vi "Filter Default message.vi"(6 "Default 3":string, 7 "new element/subarray":string[](array[string]), 8 "Default 2":string, 9 "Default 1":string, 11 "CAN TABLE":string[][](array[string])) -> (3 "CAN TABLE 2":string[][](array[string]))   [LabVIEW 2017]
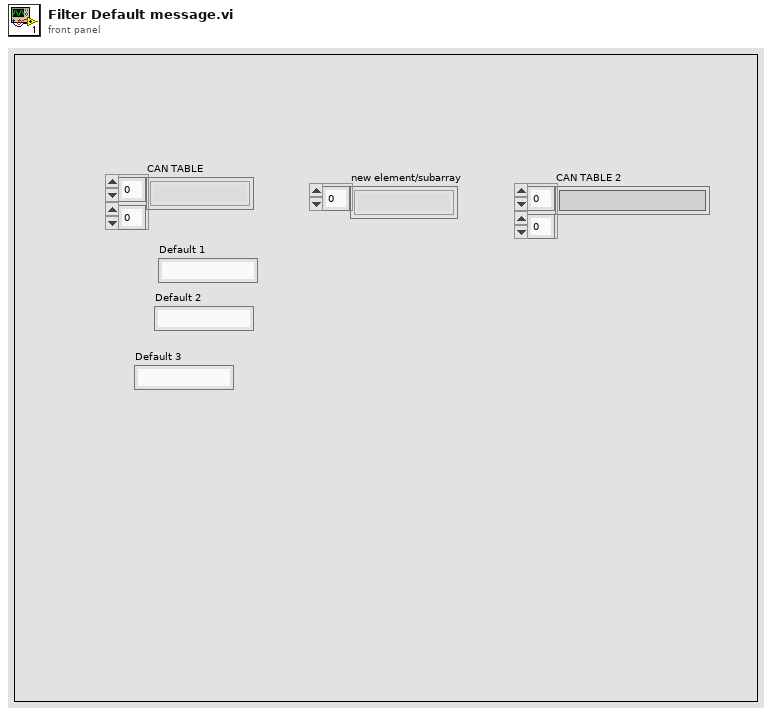
[diagram p1: front panel]
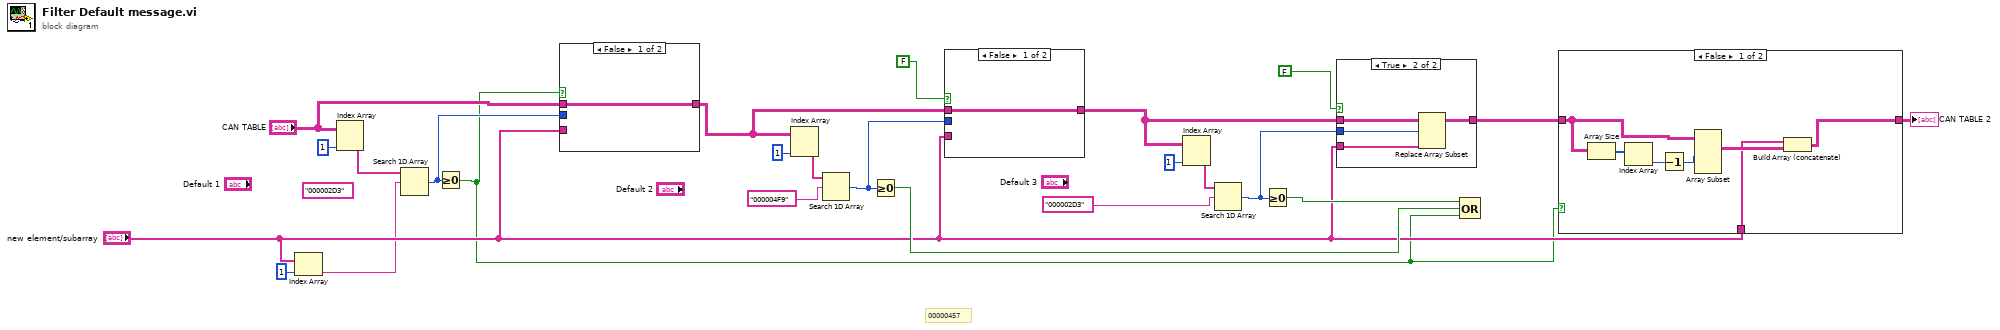
[diagram p0: block diagram]
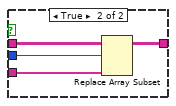
[diagram p4: hidden frame]
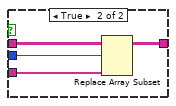
[diagram p5: hidden frame]
diagram:
  (unwired) "000002D3" ("element")
  # "00000457"
  n1 = Index Array(array="new element/subarray", index=1) -> (element=w4:string)
  n2 = Index Array(array="CAN TABLE", index (col)=1 ("disabled index (col)")) -> (element=w23:string[])  [unwired: 1 in]
  n3 = Search 1D Array(1D array=w23, element=w4) -> (index of element=w22:i32)  [unwired: 1 in]
  n4 = Greater Or Equal To 0?(x=w22) -> (x >= 0?=w1:bool)
  n5 = case shown="False" w1 {
    tunnel: w22 -> [_ w29]
    tunnel: [w25 w28] -> w18
    tunnel: "CAN TABLE" -> [w25 w27]
    tunnel: "new element/subarray" -> [_ w26]
    frame False {
    }
    frame True {
      n6 = Replace Array Subset(array=w27, new element=w26, index (row)=w29) -> (w28:string[][])  [unwired: 1 in]
    }
  }
  n7 = Index Array(array=w18, index (col)=1 ("disabled index (col)")) -> (element=w20:string[])  [unwired: 1 in]
  n8 = Search 1D Array(1D array=w20, element="000004F9") -> (index of element=w17:i32)  [unwired: 1 in]
  n9 = Greater Or Equal To 0?(x=w17) -> (x >= 0?=w11:bool)
  n10 = case shown="False" FALSE {
    tunnel: w17 -> [_ w34]
    tunnel: [w30 w33] -> w13
    tunnel: w18 -> [w30 w32]
    tunnel: "new element/subarray" -> [_ w31]
    frame False {
    }
    frame True {
      n11 = Replace Array Subset(array=w32, new element=w31, index (row)=w34) -> (w33:string[][])  [unwired: 1 in]
    }
  }
  n12 = Index Array(array=w13, index (col)=1 ("disabled index (col)")) -> (element=w14:string[])  [unwired: 1 in]
  n13 = Search 1D Array(1D array=w14, element="000002D3") -> (index of element=w16:i32)  [unwired: 1 in]
  n14 = Greater Or Equal To 0?(x=w16) -> (x >= 0?=w12:bool)
  n15 = case shown="True" FALSE {
    tunnel: w16 -> [_ w39]
    tunnel: [w35 w38] -> w10
    tunnel: w13 -> [w35 w37]
    tunnel: "new element/subarray" -> [_ w36]
    frame False {
    }
    frame True {
      n16 = Replace Array Subset(array=w37, new element=w36, index (row)=w39) -> (w38:string[][])  [unwired: 1 in]
    }
  }
  n17 = Compound Arithmetic op=OR(w12, w11, w1) -> ()  [unwired: 1 out]
  n18 = case shown="False" w1 {
    tunnel: w10 -> [w42 w47]
    tunnel: [w40 w47] -> w9
    tunnel: "new element/subarray" -> [w41 _]
    frame False {
      n19 = Array Size(array=w42) -> (size(s)=w43:i32[])
      n20 = Index Array(array=w43) -> (element=w44:i32)  [unwired: 1 in]
      n21 = Decrement(x=w44) -> (x-1=w45:i32)
      n22 = Array Subset(array=w42, length (row)=w45) -> (w46:string[][])  [unwired: 3 in]
      n23 = Build Array (concatenate)(w41, w46) -> (w40:string[][])
    }
    frame True {
    }
  }
  "CAN TABLE 2" <- w9
